vi "TCP_NoDelay_Linux.vi"(4 "error in (no error)":errorcluster, 6 "TCP_NODELAY (true)":bool=TRUE, 7 "connID":refnum<k5>) -> (0 "error out":errorcluster, 3 "connID 2":refnum<k5>)   [LabVIEW 2016]
doc: "This VI takes a LabVIEW TCP Connection ID and either sets or clears the TCP_NODELAY flag on the underlying socket. Upon creation of a socket this flag is by default clear, meaning that the Nagle algorithm is in effect. By setting the TCP_NODELAY flag, the Nagle algorithm is disabled for the given connection. \n\nYou should disable the Nagle algorithm with care - it is one of the basic algorithms of TCP that helps reduce internet traffic by coalescing several small packets into a single large one. However, sometimes disabling it is useful in reducing latency in protocols that have a query/response nature.\n\nFor more information on the Nagle algorithm, google \"nagle\".\nFor platform specific notes, see the diagram."
uses:
  libc.so.6
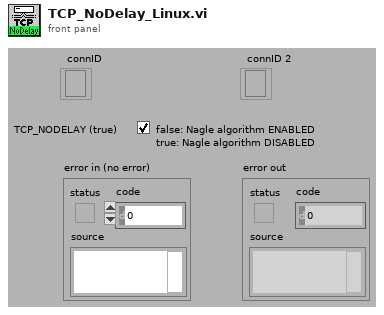
[diagram p1: front panel]
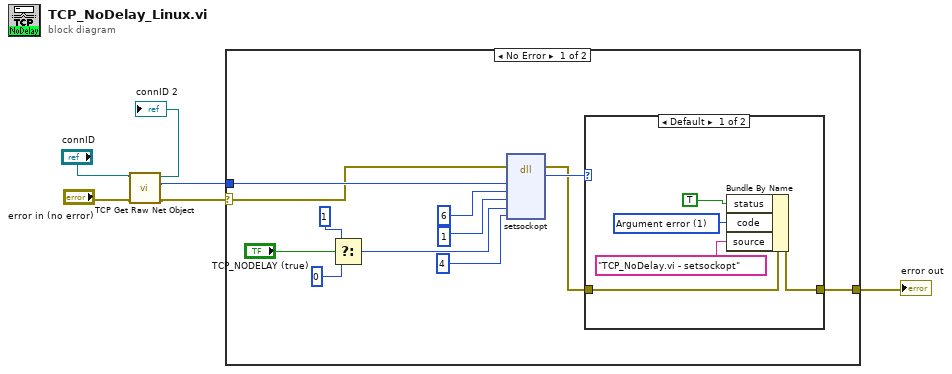
[diagram p0: block diagram]
diagram:
  n1 = call <vilib>:"TCP Get Raw Net Object.vi"("error in (no error)"="error in (no error)", "connection ID"="connID") -> ("error out"=w4:errorcluster, "raw net object"=w3:u64, "connection ID out"=→"connID 2":refnum<k5>)  [unwired: 7 in]
  n2 = case shown="No Error" w4 {
    selector: w4 -> [w10 w25]
    tunnel: [w15 w25] -> w6
    tunnel: w3 -> [w12 _]
    frame No Error {
      n3 = Select(t=1, s="TCP_NODELAY (true)", f=0) -> (s? t:f=w11:i32)
      n4 = dll-call lib="libc.so.6" fn="setsockopt"(error in=w10, "sockfd"=w12, "level"=6 ("IPPROTO"), "optname"=1 ("IPPROTO"), "optval"=w11, "optlen"=4 ("IPPROTO")) -> (error out=w9:errorcluster, "return"=w13:i32)  [unwired: 7 in, 1 out]
      n5 = case shown="Default" w13 {
        tunnel: [w23 w24] -> w15
        tunnel: w9 -> [w19 w24]
        frame Default {
          w22 = 1 items=["No error", "Argument error", "Memory is full", "Out of zone", "End of file", "File already open", "Generic file I/O error", "File not found", "File permission error", "Disk is full", "Duplicate path", "Too many files open", "System feature not enabled", "Resource file not found", "Cannot add resource", "Resource not found", "Image not found", "Image memory error", "Pen does not exist", "Config type invalid", "Config token not found", "Config parse error", "Config memory error", "Bad external code format", "Bad external code offset", "External code not present", "Null window", "Destroy window error", "Null menu", "Print aborted", "Bad print record", "Print driver error", "Windows error during printing", "Memory error during printing", "Print dialog error", "Generic print error", "Invalid device refnum", "Device not found", "Device parameter error", "Device unit error", "Cannot open device", "Device call aborted", "Generic error", "Cancelled by user", "Object ID too low", "Object ID too high", "Object not in heap", "Unknown heap", "Unknown object (invalid DefProc)", "Unknown object (DefProc not in table)", "Message out of range", "Invalid (null) method", "Unknown message", "Manager call not supported", "Bad address", "Network operation in progress", "Network operation timed out", "Connection is busy", "Network attribute not supported", "Network error", "Address in use", "System out of memory", "Connection aborted", "Connection refused", "Not connected", "Already connected", "Connection closed", "Initialization error (interapplication manager)", "Bad occurrence", "Wait on unbound occurrence handler", "Occurrence queue overflow", "Datalog type conflict", "Unused", "Unrecognized type (interapplication manager)", "Memory corrupt", "Failed to make temporary DLL", "Old CIN version", "Drag socket not found", "Failed to load drop-object", "Failed to register OLE object", "Failed to release OLE object", "Format specifier type mismatch", "Unknown format specifier", "Too few format specifiers", "Too many format specifiers", "Scan failed", "Newer CIN version", "Error converting to variant", "Runtime menu error", "Password tampered", "Variant attribute not found", "Incompatible variant data type", "Event data is not available", "Event Store is not present", "Occurrence is not found", "Event Queue is not created", "Event info is not available", "Refnum passed is NULL", "Error retrieving Class GUID", "Error retrieving CoClass GUID", "Error retrieving TypeLib GUID.", "Bad built application magic bytes.", "Specific driver is different from the specific driver associated with the Logical Name.", "There is no session opened to the class driver.", "Max Error", "MAX - Error with config objects", "MAX - Error loading configuration", "MAX - Group not supported"]
          n6 = Bundle By Name(cluster=w19, "status"=TRUE, "code"=w22, "source"="TCP_NoDelay.vi - setsockopt") -> (w23:errorcluster)
        }
        frame 0 {
        }
      }
    }
    frame Error {
    }
  }
  "error out" <- w6
